vi "temp system.vi"() -> ()   [LabVIEW 2015]
doc: "This VI is an exercise in the LabVIEW Basics I course.\n\nYou will build the diagram for this VI so that it runs as a user-driven interface. When the user presses a button, then the appropriate subVI will open. You will be modifying the SubVI Node Setup of the subVIs and the VI Properties of this VI."
panel:
  in  "display string":bool
  in  "stop":bool
  in  "Display Logged Temp":bool
  in  "Display & Log Temp":bool
  in  "Display Temp":bool
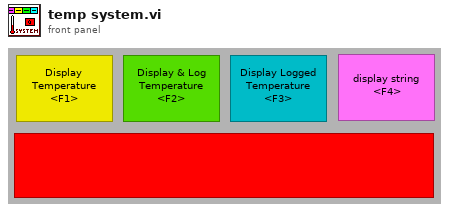
[diagram p1: front panel]
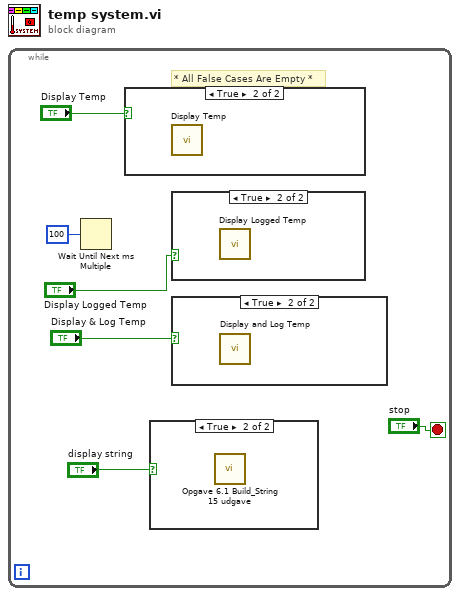
[diagram p0: block diagram]
diagram:
  n1 = while {
    stop <- "stop" stop-if-true
    # "* All False Cases Are Empty *"
    n2 = Wait Until Next ms Multiple(millisecond multiple=u32 100) -> ()  [unwired: 1 out]
    n3 = case shown="True" "Display Temp" {
      frame False {
      }
      frame True {
        n4 = call "Display Temp.vi"() -> ()  [unwired: 1 in]
      }
    }
    n5 = case shown="True" "display string" {
      frame False {
      }
      frame True {
        n6 = call "Opgave 6.1 Build_String 15 udgave.vi"() -> ()  [unwired: 8 in, 4 out]
      }
    }
    n7 = case shown="True" "Display Logged Temp" {
      frame False {
      }
      frame True {
        n8 = call "Display Logged Temp.vi"() -> ()  [unwired: 1 in]
      }
    }
    n9 = case shown="True" "Display & Log Temp" {
      frame False {
      }
      frame True {
        n10 = call "Display and Log Temp.vi"() -> ()  [unwired: 1 in]
      }
    }
  }
